vi "Learning coeff (SubVI).vi"(11 "file path (use dialog)":path) -> (2 "initialized array":dbl[](array[numeric]), 3 "path":path)   [LabVIEW 2025]
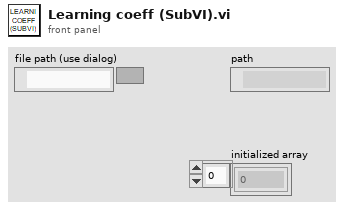
[diagram p1: front panel]
types:
  T1 = enum16{"open", "replace", "create", "open or create", "replace or create", "replace or create with confirmation"}
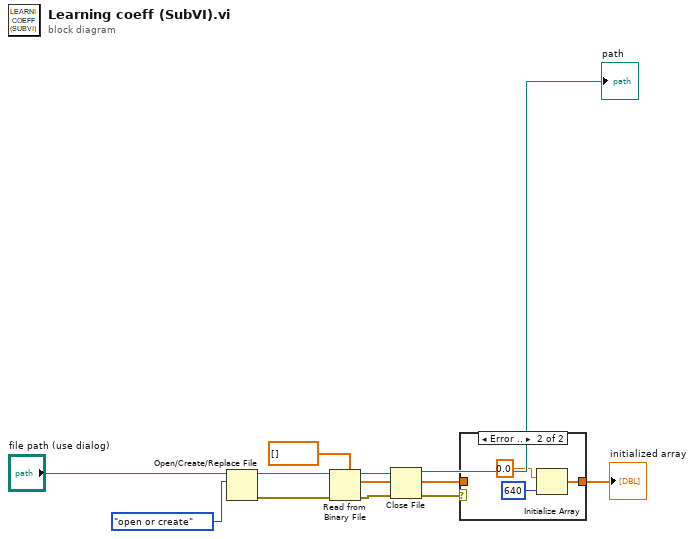
[diagram p0: block diagram]
diagram:
  n1 = Open/Create/Replace File(file path (use dialog)="file path (use dialog)", operation (0:open)=T1."open or create") -> (refnum out=w4:refnum<file>, error out=w5:errorcluster)  [unwired: 4 in, 1 out]
  n2 = Read from Binary File(5:dbl[] [] ("initialized array"), 8:w5, 11:w4) -> (0:w10:errorcluster, 2:w7:dbl[], 3:w8:refnum<file>)  [unwired: 3 in, 1 out]
  n3 = Close File(refnum=w8, error in=w10) -> (path=→"path":path, error out=w11:errorcluster)
  n4 = case shown="Error .." w11 {
    tunnel: [w12 w14] -> w3
    tunnel: w7 -> [w12 _]
    frame No Error {
    }
    frame Error {
      n5 = Initialize Array(0.0 ("element"), 640 ("dimension size")) -> (w14:dbl[])
    }
  }
  "initialized array" <- w3
